vi "Exchange Param.vi"(8 "error in (no error)":errorcluster, 9 "PAR in":dbl[](array[numeric]), 10 "PAR_I in":i32[](array[numeric]), 11 "PAR DVR":refnum<data-value>) -> (0 "error out":errorcluster, 1 "PAR out":dbl[](array[numeric]), 2 "PAR_I out":i32[](array[numeric]), 3 "PAR DVR out":refnum<data-value>)   [LabVIEW 2019, in "Inputs.lvlib"]
uses:
  Inputs.lvlib
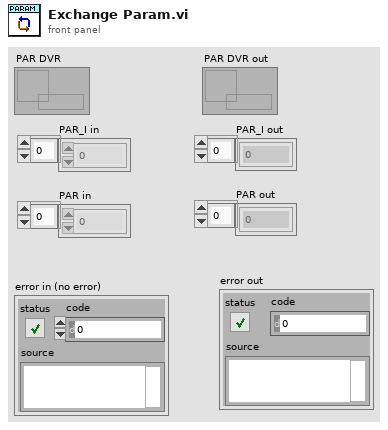
[diagram p1: front panel]
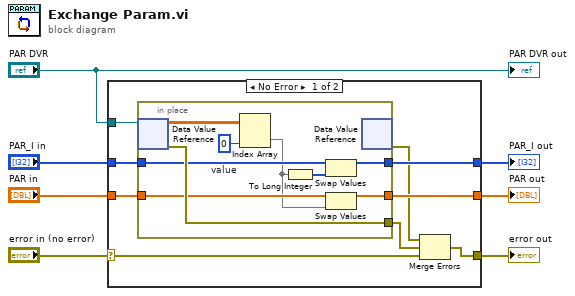
[diagram p0: block diagram]
diagram:
  n1 = case shown="No Error" "error in (no error)" {
    selector: "error in (no error)" -> [w8 w26]
    tunnel: [w16 w27] -> w7
    tunnel: "PAR in" -> [w15 w27]
    tunnel: [w14 w28] -> w5
    tunnel: "PAR_I in" -> [w13 w28]
    tunnel: "PAR DVR" -> [w12 _]
    tunnel: [w9 w26] -> w3
    frame No Error {
      n2 = in-place {
        in-place-border: [w25] -> w10
        in-place-border: w13 -> [w22]
        in-place-border: [w21] -> w14
        in-place-border: w15 -> [w19]
        in-place-border: [w18] -> w16
        w24 = 0  # value
        n3 = in-place-dvr #1(w12) -> (w23:dbl[][], w25:errorcluster)
        n4 = Index Array(array=w23, index (col)=w24) -> (element=w17:dbl[])  [unwired: 1 in]
        n5 = To Long Integer(number=w17) -> (32bit integer=w20:i32[])
        n6 = Swap Values(12:w22, 14:w20) -> (1:w21:i32[])  [unwired: 1 in, 1 out]
        n7 = Swap Values(12:w19, 14:w17) -> (1:w18:dbl[])  [unwired: 1 in, 1 out]
        n8 = in-place-dvr #1() -> (w11:errorcluster)  [unwired: 1 in, 1 out]
      }
      n9 = Merge Errors(w11, w10, w8) -> (w9:errorcluster)
    }
    frame Error {
    }
  }
  "PAR out" <- w7
  "PAR_I out" <- w5
  "error out" <- w3
  "PAR DVR out" <- "PAR DVR"
